vi "Get Slope and Intercept.vi"(10 "Read Dark File":dbl[](array[numeric]), 11 "Integration Time":sgl) -> (2 "Intercept Out":dbl, 3 "Slope Out":dbl)   [LabVIEW 2014, in "AvaSpec.lvlib" / "Dark.lvlib"]
doc: "Parses the slope and intercept values from the dark model file"
uses:
  <vilib>/express/express arith-compare/Formula/XNode/ExpressFormulaBlockNode.xnode
  Dark.lvlib
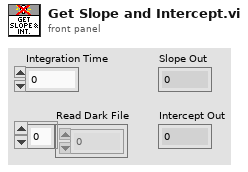
[diagram p1: front panel]
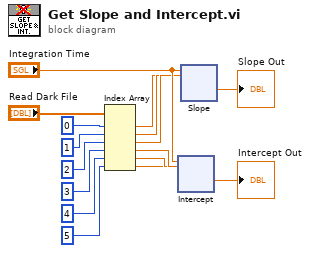
[diagram p0: block diagram]
diagram:
  n1 = Index Array(array="Read Dark File", index #1=0 ("index"), index #2=1 ("index"), index #3=2 ("index"), index #4=3 ("index"), index #5=4 ("index"), index #6=5 ("index")) -> (element #1=w7:dbl, element #2=w8:dbl, element #3=w9:dbl, element #4=w12:dbl, element #5=w11:dbl, element #6=w10:dbl)
  n2 = xnode "Intercept"("intTime"="Integration Time", "a"=w12, "b"=w11, "c"=w10) -> ("Result"=→"Intercept Out":dbl)  [unwired: 1 in, 1 out]
  n3 = xnode "Slope"("intTime"="Integration Time", "a"=w7, "b"=w8, "c"=w9) -> ("Result"=→"Slope Out":dbl)  [unwired: 1 in, 1 out]
